vi "Configuration Name--constant.vi"() -> (3 "Configuration Name":string)   [LabVIEW 2020, in "Performance Monitor UI.lvlib" / "Configuration.lvlib"]
doc: "Configuration name. This name is used when registering the module configuration with the DCFG Framework. Make sure you don't hard code this anywhere, and always use this VI when referring to the configuration or its pages.\n_____\nBased on DCFG Project Template 1.0.0.21.\n____\nPeloton Config 1.0.0.2\nCopyright (c) 2022, Peloton"
uses:
  Configuration.lvlib
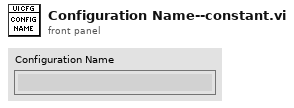
[diagram p1: front panel]
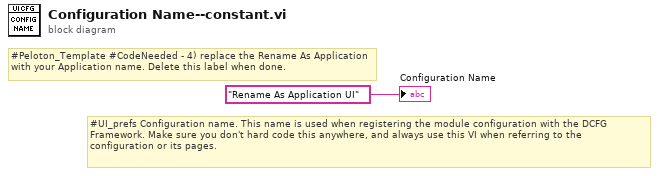
[diagram p0: block diagram]
diagram:
  # "#Peloton_Template #CodeNeeded - 4) replace the Rename As Application with your Application name. Delete this label when done."
  # "#UI_prefs Configuration name. This name is used when registering the module configuration with the DCFG Framework. Make sure you don't hard code this anywhere, and always use this VI when referring to the configuration or its pages."
  "Configuration Name" <- "Rename As Application UI" ("Configuration Name")
